vi "Labspec GetValueSimple.vi"(6 "Variable Type":u16(ring) items=["Integer"=3, "Float"=4, "Double"=5, "Byte"=17], 8 "error in":errorcluster, 9 "Acquisition Mode":u16(ring) items=["XY Data", "Data", "Axis Labels", "Axis Units", "Axis", "Axis Index", "Axis Size", "Axis Type", "Intensity", "Frequency", "X", "Y", "Z", "Time"], 10 "DataID":i32, 11 "Automation Refnum In":refnum<k7>) -> (0 "error out":errorcluster, 1 "pValue":variant, 3 "Automation Refnum Out":refnum<k7>)   [LabVIEW 2014]
panel:
  out "Value":dbl
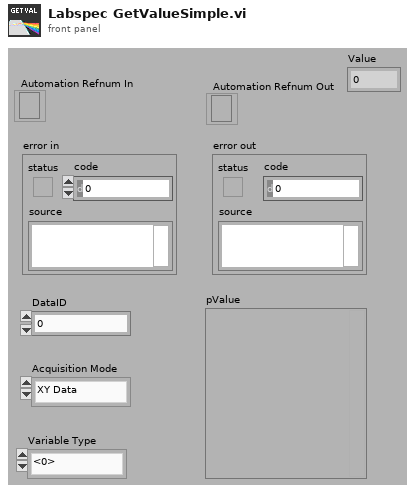
[diagram p1: front panel]
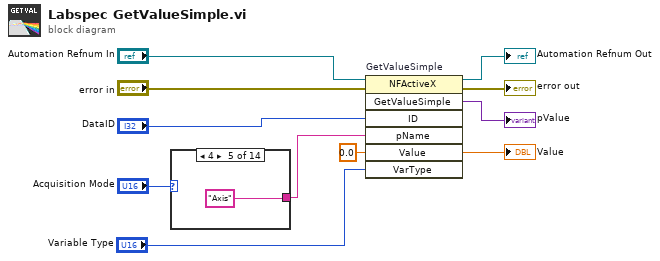
[diagram p0: block diagram]
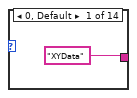
[diagram p2: hidden frame]
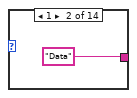
[diagram p3: hidden frame]
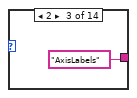
[diagram p4: hidden frame]
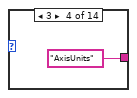
[diagram p5: hidden frame]
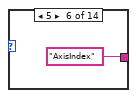
[diagram p6: hidden frame]
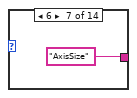
[diagram p7: hidden frame]
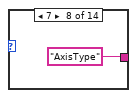
[diagram p8: hidden frame]
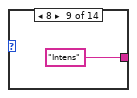
[diagram p9: hidden frame]
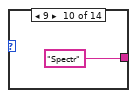
[diagram p10: hidden frame]
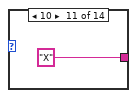
[diagram p11: hidden frame]
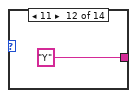
[diagram p12: hidden frame]
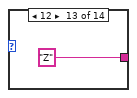
[diagram p13: hidden frame]
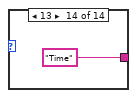
[diagram p14: hidden frame]
diagram:
  n1 = case shown="4" "Acquisition Mode" {
    tunnel: ["XYData" "Data" "AxisLabels" "AxisUnits" "Axis" "AxisIndex" "AxisSize" "AxisType" "Intens" "Spectr" "X" "Y" "Z" "Time"] -> w6
    frame 0, Default {
    }
    frame 1 {
    }
    frame 2 {
    }
    frame 3 {
    }
    frame 4 {
    }
    frame 5 {
    }
    frame 6 {
    }
    frame 7 {
    }
    frame 8 {
    }
    frame 9 {
    }
    frame 10 {
    }
    frame 11 {
    }
    frame 12 {
    }
    frame 13 {
    }
  }
  n2 = invoke on="GetValueSimple" class="NFActiveX" method="GetValueSimple"(reference="Automation Refnum In", error in="error in", "ID"="DataID", "pName"=w6, "Value"=0.0, "VarType"="Variable Type") -> (reference out=→"Automation Refnum Out":refnum<k7>, error out=→"error out":errorcluster, "GetValueSimple"=→"pValue":variant, "Value"=→"Value":dbl)  [unwired: 1 in, 3 out]
